vi "Parse-Add_Scans.vi"(9 "Wall Thickness":i32, 11 "Existing Indices In":T1[](array[typedef])) -> (3 "Indices With Scan":T1[](array[typedef]))   [LabVIEW 2020]
doc: "<B>Description:</B> Adds the Lines that were actually scanned to the Indices Array and sets the Lines that were used to find the Line to scan to be not scanned.\n\n<B>Date:</B> 06/2019\n<B>Author:</B> Luke Jarocki, Choose Movement Consulting, LLC"
uses:
  Controls/Scan_Values.ctl
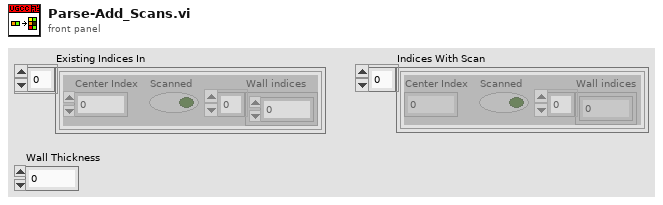
[diagram p1: front panel]
types:
  T1 = typedef "Scan_Values.ctl" = cluster{"Center Index":i32, "Scanned":bool, "Wall indices":i32[]}
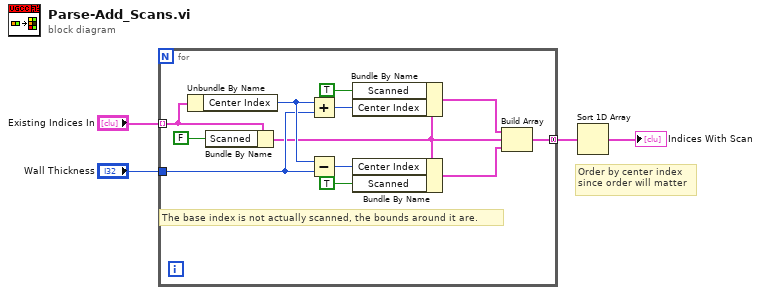
[diagram p0: block diagram]
diagram:
  # "Order by center index\nsince order will matter"
  n1 = for {
    tunnel: "Existing Indices In" -> [w7] mode=indexing
    tunnel: [w16] -> w2 mode=concatenating
    tunnel: "Wall Thickness" -> [w9]
    # "The base index is not actually scanned, the bounds around it are."
    n2 = Unbundle By Name(w7) -> ("Center Index"=w15:i32)
    n3 = Bundle By Name(cluster=w7, "Scanned"=FALSE) -> (w5:T1)
    n4 = Add(x=w15, y=w9) -> (x+y=w14:i32)
    n5 = Subtract(x=w15, y=w9) -> (x-y=w13:i32)
    n6 = Bundle By Name(cluster=w5, "Scanned"=TRUE, "Center Index"=w14) -> (w11:T1)
    n7 = Bundle By Name(cluster=w5, "Center Index"=w13, "Scanned"=TRUE) -> (w12:T1)
    n8 = Build Array(w11, w5, w12) -> (w16:T1[])
  }
  n9 = Sort 1D Array(array=w2) -> (sorted array=→"Indices With Scan":T1[])
